vi "State_Machine.vi"(8 "error in (no error)":errorcluster caption="entrée d'erreur (pas d'erreur)", 11 "Delay en entrée":refnum<class "Ask_Loop_Group.lvclass">) -> (0 "error out":errorcluster caption="sortie d'erreur", 2 "Json_String":string, 3 "Delay en sortie":refnum<class "Ask_Loop_Group.lvclass">)   [LabVIEW 2020, in "Library Test.lvlib" / "Ask_Loop_Group.lvclass"]
uses:
  Ask_Loop_Group.lvclass
  C:/Users/ngarcin/OneDrive - Altyor/Standard TB/Suite TB45/Class/Test/Test (Default)/Test (Default).lvclass
  Commun VI/TypeDef/Variable Printable.ctl
  JSON API/JSON Value/Set from JSON string.vi
  JSON API/JSON Value/JSON Value.lvclass
  JSON API/Variant JSON/Variant JSON.lvlib
  JSON API/Get Polymorphic/JSON GetSet.lvlib
  Commun VI/Library Commun.lvlib
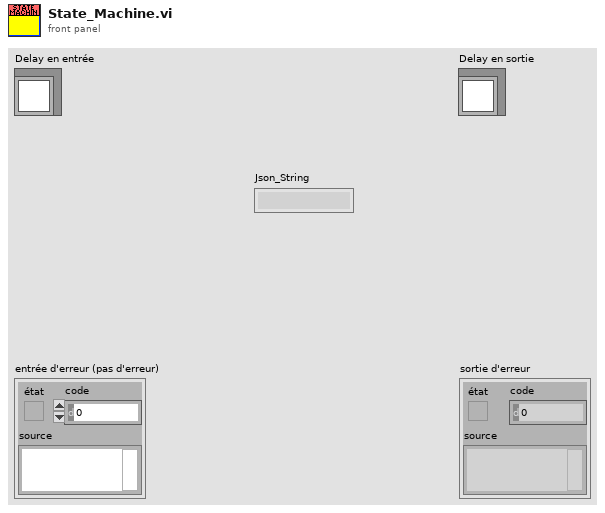
[diagram p1: front panel]
types:
  T1 = typedef "Variable Printable.ctl" = string
  T2 = enum16{"Get Variable", "Get All Variables", "Set Variable", "Delete Variable", "Delete All Variable"}
  T3 = enum16{"Get Loop Sequence", "Reset", "Set Loop Sequence"}
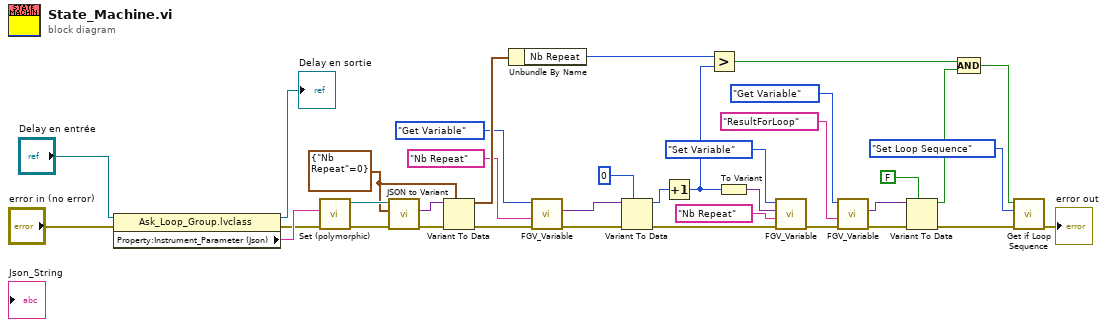
[diagram p0: block diagram]
diagram:
  w24 = cluster{"Nb Repeat":i32} {"Nb Repeat"=0}
  n1 = property class="Ask_Loop_Group.lvclass"(reference="Delay en entrée", error in="error in (no error)") -> (reference out=→"Delay en sortie":refnum<class "Ask_Loop_Group.lvclass">, error out=w28:errorcluster, "Property:Instrument_Parameter (Json)"=w31:string)
  n2 = call-poly "Set (polymorphic).vi"("error in (no error)"=w28, "JSON stream"=w31) -> ("error out"=w33:errorcluster, "JSON Value out"=w35:refnum<class "JSON Value.lvclass">)  [unwired: 7 in, 1 out]
  n3 = call "JSON to Variant.vi"("error in (no error)"=w33, "Variant (Data Type)"=w24, "JSON Value"=w35) -> ("error out"=w34:errorcluster, "Variant out"=w32:variant)  [unwired: 7 in]
  n4 = Variant To Data(error in=w34, type=w24, Variant=w32) -> (data=w25:cluster{"Nb Repeat":i32}, error out=w14:errorcluster)
  n5 = Unbundle By Name(w25) -> ("Nb Repeat"=w4:i32)
  n6 = call "FGV_Variable.vi"("error in (no error)"=w14, "Variable"=T1 "Nb Repeat", "Function"=T2."Get Variable") -> ("error out"=w15:errorcluster, "Data Out"=w13:variant)  [unwired: 6 in, 1 out]
  n7 = Variant To Data(error in=w15, type=0, Variant=w13) -> (data=w12:i32, error out=w11:errorcluster)
  n8 = Increment(x=w12) -> (x+1=w5:i32)
  n9 = Greater?(x=w4, y=w5) -> (0:w3:bool)
  n10 = To Variant(anything=w5) -> (Variant=w17:variant)
  n11 = call "FGV_Variable.vi"("error in (no error)"=w11, "Variable"=T1 "Nb Repeat", "Data In"=w17, "Function"=T2."Set Variable") -> ("error out"=w7:errorcluster)  [unwired: 5 in, 2 out]
  n12 = call "FGV_Variable.vi"("error in (no error)"=w7, "Variable"=T1 "ResultForLoop", "Function"=T2."Get Variable") -> ("error out"=w10:errorcluster, "Data Out"=w8:variant)  [unwired: 6 in, 1 out]
  n13 = Variant To Data(error in=w10, type=FALSE, Variant=w8) -> (data=w6:bool, error out=w1:errorcluster)
  n14 = Compound Arithmetic op=AND ("Opérateur arithmétique")(w3, w6) -> (w2:bool)
  n15 = call "Get if Loop Sequence.vi"("error in (no error)"=w1, "Function"=T3."Set Loop Sequence", "Loop In"=w2) -> ("error out"=→"error out":errorcluster)  [unwired: 7 in, 1 out]
